vi "PhotonTrackedTarget_GetCorners.vi"(11 "TrackedTarget":T2={"Yaw"=0.0, "Pitch"=0.0, "Area"=0.0, "Skew"=0.0, "TargetCorners"=[], "BestCameraToTarget"={"TRANSLATION"={"X"=0.0, "Y"=0.0}, "ROTATION"={"VALUE"=0.0, "COS"=1.0, "SIN"=0.0}, "xF"=FALSE}, "FiducialId"=0, "AltCameraToTarget"={"TRANSLATION"={"X"=0.0, "Y"=0.0}, "ROTATION"={"VALUE"=0.0, "COS"=1.0, "SIN"=0.0}, "xF"=FALSE}, "Ambiguity"=0.0} {"AltCameraToTarget"."ROTATION"."SIN" format="%13.4f"; "AltCameraToTarget"."ROTATION"."COS" format="%13.4f"; "AltCameraToTarget"."ROTATION"."VALUE" format="%13.4f"; "AltCameraToTarget"."TRANSLATION"."Y" format="%14.3f"; "AltCameraToTarget"."TRANSLATION"."X" format="%14.3f"; "BestCameraToTarget"."ROTATION"."SIN" format="%13.4f"; "BestCameraToTarget"."ROTATION"."COS" format="%13.4f"; "BestCameraToTarget"."ROTATION"."VALUE" format="%13.4f"; "BestCameraToTarget"."TRANSLATION"."Y" format="%14.3f"; "BestCameraToTarget"."TRANSLATION"."X" format="%14.3f"}) -> (3 "TargetCorners":T1[](array[typedef]))   [LabVIEW 2020, in "PhotonVisionLib.lvlib"]
doc: "Get Corners from Tracked Target\n\nInputs:\n - TrackedTarget -- Parsed TrackedTarget cluster.\n\nOutputs:\n - Corners -- Corners array of TargetCorner cluster"
uses:
  PhotonVisionLib.lvlib
  TypeDef/PhotonTrackedTargetType.ctl
  TypeDef/TargetCornerType.ctl
  <vilib>/Rock Robotics/WPI/ThirdParty/JAS_Junk/TrajLib/TypeDef/TRANSFORM2D.ctl
  <vilib>/Rock Robotics/WPI/ThirdParty/JAS_Junk/TrajLib/TypeDef/TRANSLATION2D.ctl
  <vilib>/Rock Robotics/WPI/ThirdParty/JAS_Junk/TrajLib/TypeDef/ROTATION2D.ctl
  <vilib>/Rock Robotics/WPI/ThirdParty/JAS_Junk/TrajLib/Trajectory_Library.lvlib
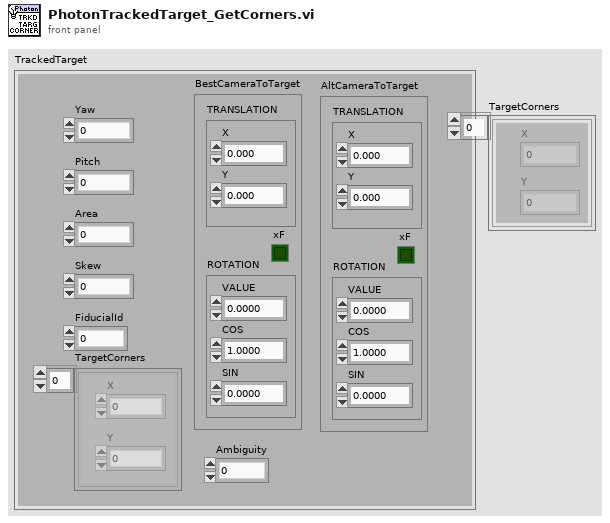
[diagram p1: front panel]
types:
  T1 = typedef "PhotonVisionLib.lvlib/TargetCornerType.ctl" = cluster{"X":dbl, "Y":dbl}
  T2 = typedef "PhotonVisionLib.lvlib/PhotonTrackedTargetType.ctl" = cluster{"Yaw":dbl, "Pitch":dbl, "Area":dbl, "Skew":dbl, "TargetCorners":T1[], "BestCameraToTarget":T3, "FiducialId":i32, "AltCameraToTarget":T3, "Ambiguity":dbl}
  T3 = typedef "Trajectory_Library.lvlib/TRANSFORM2D.ctl" = cluster{"TRANSLATION":T4, "ROTATION":T5, "xF":bool}
  T4 = typedef "Trajectory_Library.lvlib/TRANSLATION2D.ctl" = cluster{"X":dbl, "Y":dbl}
  T5 = typedef "Trajectory_Library.lvlib/ROTATION2D.ctl" = cluster{"VALUE":dbl, "COS":dbl, "SIN":dbl}
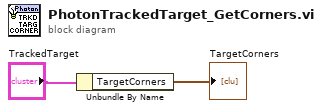
[diagram p0: block diagram]
diagram:
  n1 = Unbundle By Name("TrackedTarget") -> ("TargetCorners"=→"TargetCorners":T1[])
